vi "Simpe_IQBlock_Example_lx.vi"() -> ()   [LabVIEW 2017]
uses:
  <userlib>/RSA_API/RSA_API.lvlib
panel:
  out "qData":waveform(sgl)(graph)
  out "iData":waveform(sgl)(graph)
  out "iqOutputLength":i32
  out "iqBWOut":dbl=2445300000.0 format="%#_13g"
  out "RecordLengthOut":dbl=2445300000.0 format="%#_13g"
  out "RefLevelOut":dbl=2445300000.0 format="%#_13g"
  out "CFOut":dbl=2445300000.0 format="%#_13g"
  out "String 2":string
  out "String":string
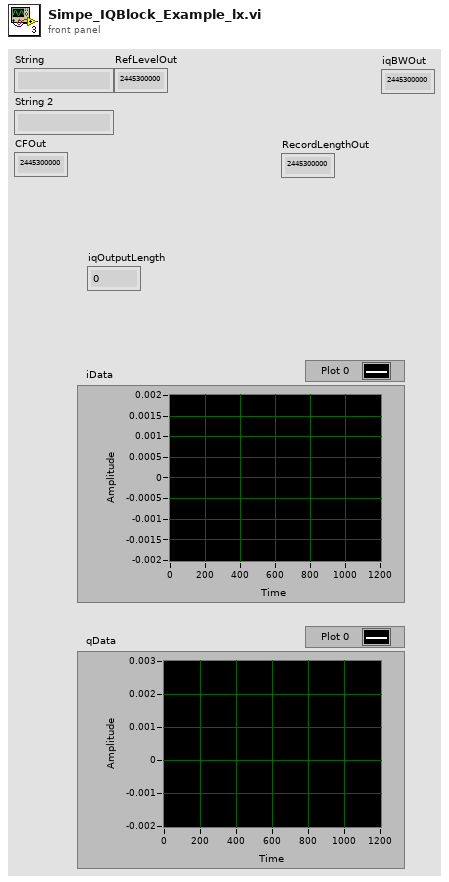
[diagram p1: front panel]
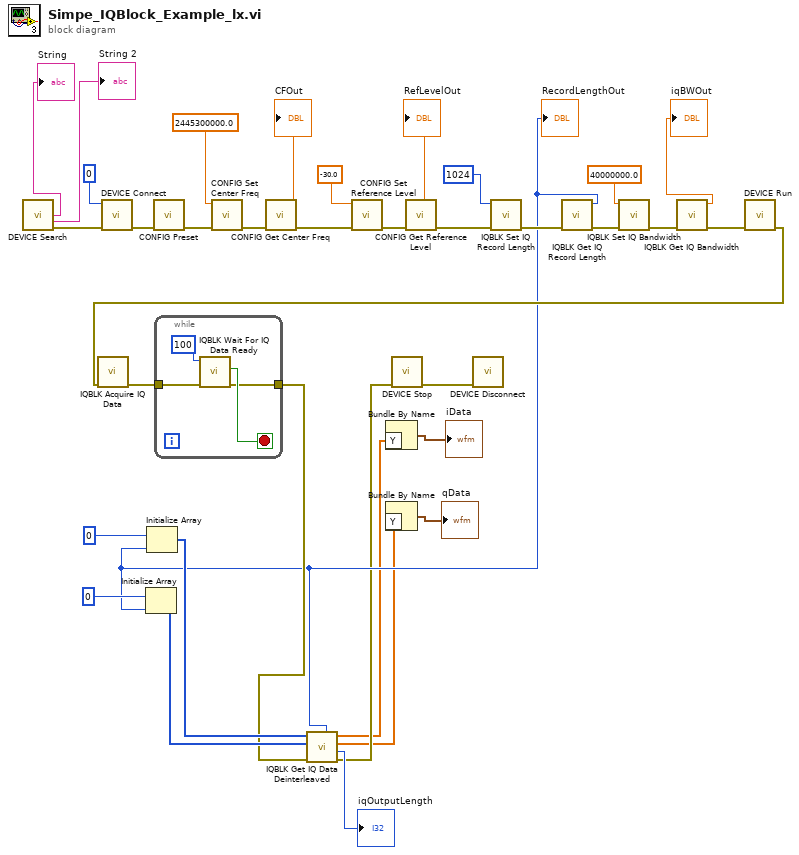
[diagram p0: block diagram]
diagram:
  n1 = call <userlib>:"DEVICE Search.vi"() -> ("deviceSerial out"=→"String":string, "deviceType out"=→"String 2":string, "error out"=w36:errorcluster)  [unwired: 10 in, 3 out]
  n2 = call <userlib>:"DEVICE Connect.vi"("error in (no error)"=w36, "deviceID"=0) -> ("error out"=w31:errorcluster)  [unwired: 8 in, 1 out]
  n3 = call <userlib>:"CONFIG Preset.vi"("error in (no error)"=w31) -> ("error out"=w30:errorcluster)  [unwired: 9 in, 1 out]
  n4 = call <userlib>:"CONFIG Set Center Freq.vi"("error in (no error)"=w30, "cf"=2445300000.0) -> ("error out"=w35:errorcluster)  [unwired: 8 in, 1 out]
  n5 = call <userlib>:"CONFIG Get Center Freq.vi"("error in (no error)"=w35) -> ("error out"=w34:errorcluster, "cf out"=→"CFOut":dbl)  [unwired: 8 in, 1 out]
  n6 = call <userlib>:"CONFIG Set Reference Level.vi"("error in (no error)"=w34, "refLevel"=-30.0 ("RefLevelIn")) -> ("error out"=w32:errorcluster)  [unwired: 8 in, 1 out]
  n7 = call <userlib>:"CONFIG Get Reference Level.vi"("error in (no error)"=w32) -> ("error out"=w22:errorcluster, "refLevel out"=→"RefLevelOut":dbl)  [unwired: 8 in, 1 out]
  n8 = call <userlib>:"IQBLK Set IQ Record Length.vi"("error in (no error)"=w22, "recordLength"=1024) -> ("error out"=w21:errorcluster)  [unwired: 8 in, 1 out]
  n9 = call <userlib>:"IQBLK Get IQ Record Length.vi"("error in (no error)"=w21) -> ("error out"=w20:errorcluster, "recordLength out"=w4:i32)  [unwired: 8 in, 1 out]
  "RecordLengthOut" <- w4
  n10 = Initialize Array(0, w4) -> (w7:i32[])
  n11 = Initialize Array(0, w4) -> (w8:i32[])
  n12 = call <userlib>:"IQBLK Set IQ Bandwidth.vi"("error in (no error)"=w20, "iqBandwidth"=40000000.0) -> ("error out"=w23:errorcluster)  [unwired: 8 in, 1 out]
  n13 = call <userlib>:"IQBLK Get IQ Bandwidth.vi"("error in (no error)"=w23) -> ("error out"=w15:errorcluster, "iqBandwidth out"=→"iqBWOut":dbl)  [unwired: 8 in, 1 out]
  n14 = call <userlib>:"DEVICE Run.vi"("error in (no error)"=w15) -> ("error out"=w14:errorcluster)  [unwired: 9 in, 1 out]
  n15 = call <userlib>:"IQBLK Acquire IQ Data.vi"("error in (no error)"=w14) -> ("error out"=w16:errorcluster)  [unwired: 9 in, 1 out]
  n16 = while {
    tunnel: w16 -> [w39]
    tunnel: [w38] -> w6
    stop <- w40 stop-if-true
    n17 = call <userlib>:"IQBLK Wait For IQ Data Ready.vi"("error in (no error)"=w39, "timeoutMsec"=100) -> ("error out"=w38:errorcluster, "ready out"=w40:bool)  [unwired: 7 in, 1 out]
  }
  n18 = call <userlib>:"IQBLK Get IQ Data Deinterleaved.vi"("iData"=w8, "qData"=w7, "error in (no error)"=w6, "reqLength"=w4) -> ("iData 2"=w2:sgl[], "qData 2"=w1:sgl[], "outLength out"=→"iqOutputLength":i32, "error out"=w3:errorcluster)  [unwired: 3 in]
  n19 = Bundle By Name("Y"=w2) -> (→"iData":waveform(sgl))  [unwired: 1 in]
  n20 = Bundle By Name("Y"=w1) -> (→"qData":waveform(sgl))  [unwired: 1 in]
  n21 = call <userlib>:"DEVICE Stop.vi"("error in (no error)"=w3) -> ("error out"=w13:errorcluster)  [unwired: 9 in, 1 out]
  n22 = call <userlib>:"DEVICE Disconnect.vi"("error in (no error)"=w13) -> ()  [unwired: 9 in, 2 out]
